vi "test Basic 64 bit.vi"(8 "error in (no error)":errorcluster, 11 "TestCase in":refnum<class "Service Name Tests.lvclass">=refnum) -> (0 "error out":errorcluster, 3 "TestCase out":refnum<class "Service Name Tests.lvclass">)   [LabVIEW 2017, in "Service Name Tests.lvclass"]
uses:
  Service Name Tests.lvclass
  CLI Class/CLI.lvclass
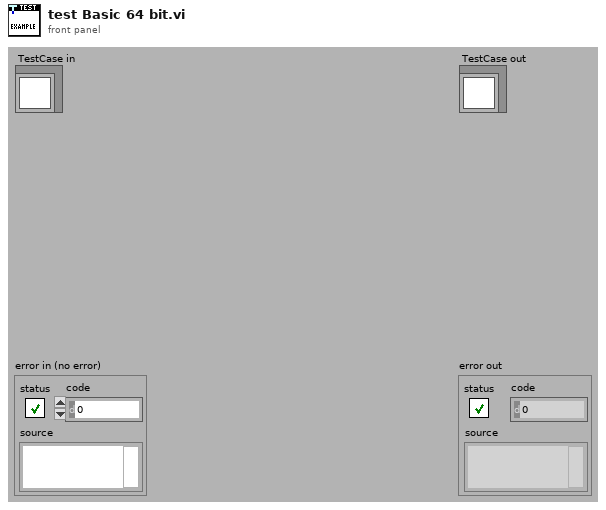
[diagram p1: front panel]
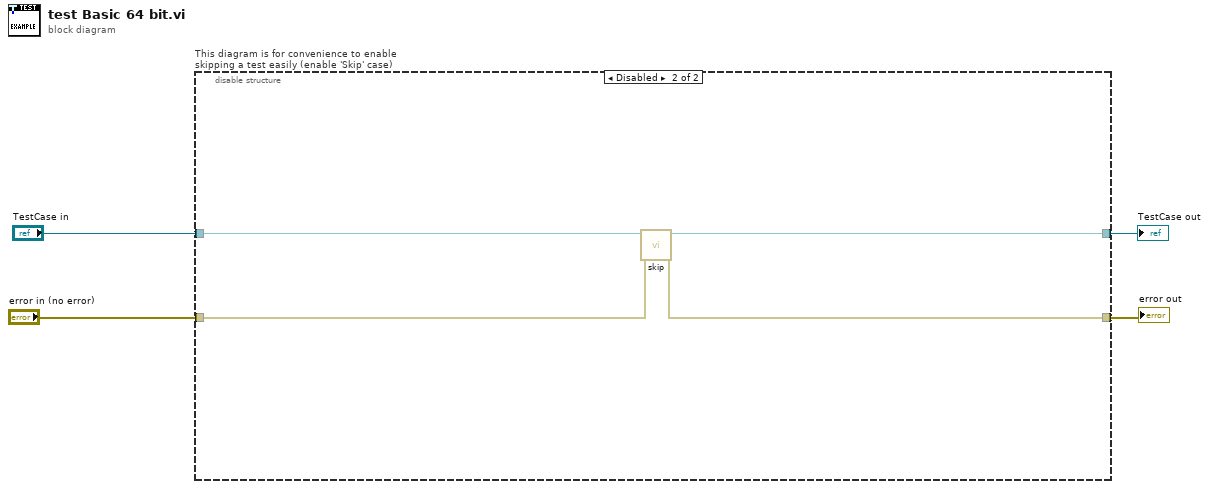
[diagram p0: block diagram]
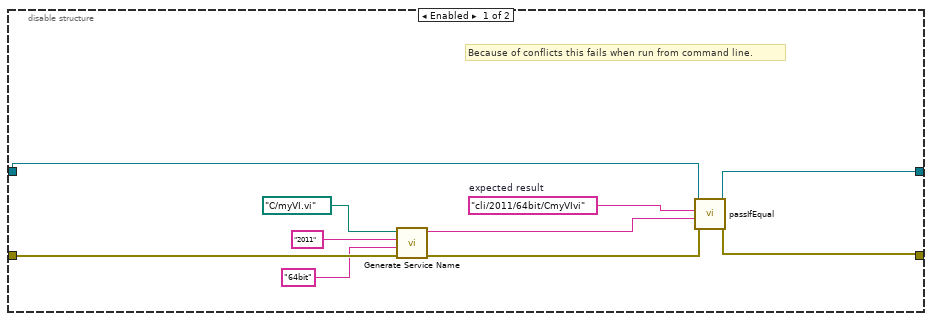
[diagram p2: hidden frame]
diagram:
  n1 = disable-structure "This diagram is for convenience to enable skipping a test easily (enable 'Skip' case)" shown="Disabled" {
    disable-tunnel: "TestCase in" -> [w13 w18]
    disable-tunnel: [w12 w16] -> w1
    disable-tunnel: [w11 w17] -> w3
    disable-tunnel: "error in (no error)" -> [w10 w15]
    frame Enabled {
      w14 = "cli/2011/64bit/CmyVIvi"  # expected result
      # "Because of conflicts this fails when run from command line."
      n2 = call "Generate Service Name.vi"("error in (no error)"=w10, "Bitness Text"="64bit", "LV Version"="2011", "VI Path"=path "C:/myVI.vi") -> ("error out"=w9:errorcluster, "Service Name"=w8:string)  [unwired: 6 in]
      n3 = call-dynamic "passIfEqual.vi"("error in (no error)"=w9, "y"=w8, "x"=w14, "TestCase in"=w13) -> ("error out"=w11:errorcluster, "TestCase out"=w12:refnum<class "Service Name Tests.lvclass">)  [unwired: 6 in]
    }
    frame Disabled {
      n4 = call <vilib>:"skip.vi"("error in (no error)"=w15, "TestCase in"=w18) -> ("error out"=w17:errorcluster, "TestCase out"=w16:refnum<class "Service Name Tests.lvclass">)  [unwired: 8 in]
    }
  }
  "error out" <- w3
  "TestCase out" <- w1
